vi "Configure Math (Binary Operation).vi"(0 "VISA resource name":refnum<visa-resource-name>, 1 "Enable Math Channel (T:Enable)":bool=TRUE, 2 "Math Operation (12: Add)":i32(ring)=12 items=["Add"=12, "Divide"=13, "Multiply"=14, "Subtract"=15, "Common Mode"=16, "Versus"=17], 5 "Math Channel (0: Function 1)":i32(ring) items=["Function 1", "Function 2", "Function 3", "Function 4", "Function 5", "Function 6", "Function 7", "Function 8", "Function 9", "Function 10", "Function 11", "Function 12", "Function 13", "Function 14", "Function 15", "Function 16"], 7 "Math Operand (1: Channel 1)":i32(ring)=1 items=["Channel 1"=1, "Channel 2"=2, "Channel 3"=3, "Channel 4"=4, "Function 1"=5, "Function 2"=6, "Function 3"=7, "Function 4"=8, "Memory 1"=9, "Memory 2"=10, "Memory 3"=11, "Memory 4"=12, "Differential 1"=61, "Differential 2"=62, "Common 1"=71, "Common 2"=72], 9 "Math Operand 2 (2: Channel 2)":i32(ring)=2 items=["Channel 1"=1, "Channel 2"=2, "Channel 3"=3, "Channel 4"=4, "Function 1"=5, "Function 2"=6, "Function 3"=7, "Function 4"=8, "Memory 1"=9, "Memory 2"=10, "Memory 3"=11, "Memory 4"=12, "Differential 1"=61, "Differential 2"=62, "Common 1"=71, "Common 2"=72], 11 "error in (no error)":errorcluster) -> (4 "VISA resource name out":refnum<visa-resource-name>, 15 "error out":errorcluster)   [LabVIEW 2020, in "Agilent 90000 Series.lvlib"]
doc: "Creates a mathematical expression with two operands."
uses:
  Agilent 90000 Series.lvlib
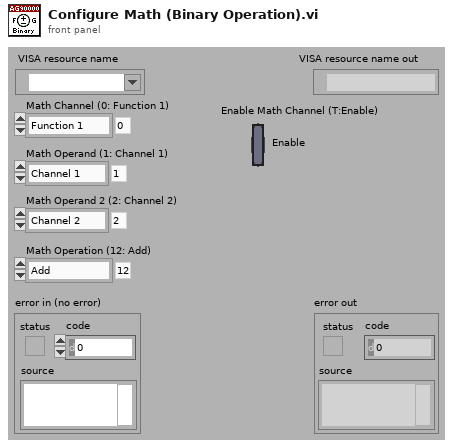
[diagram p1: front panel]
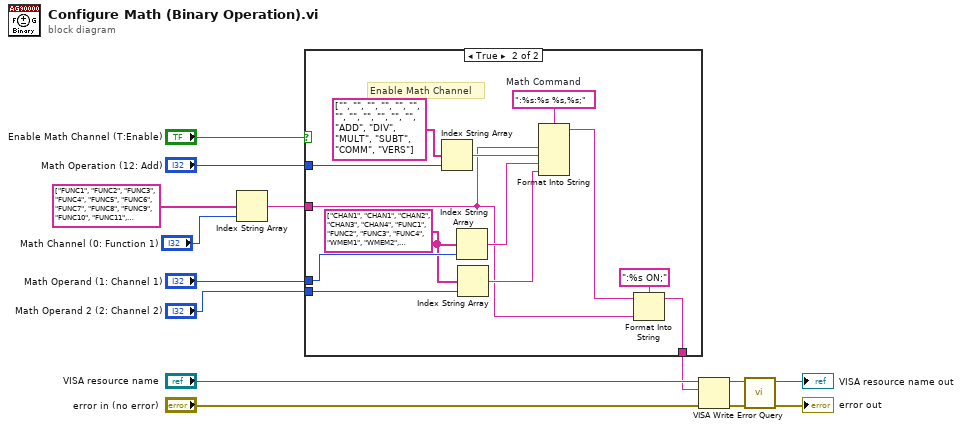
[diagram p0: block diagram]
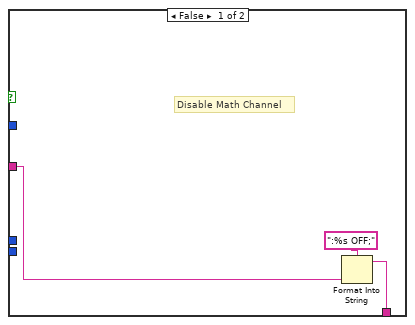
[diagram p2: hidden frame]
diagram:
  n1 = Index String Array(1:"Math Channel (0: Function 1)", 2:string[] ["FUNC1", "FUNC2", "FUNC3", "FUNC4", "FUNC5", "FUNC6", "FUNC7", "FUNC8", "FUNC9", "FUNC10", "FUNC11", "FUNC12", "FUNC13", "FUNC14", "FUNC15", "FUNC16"] ("string array")) -> (0:w7:string)  [unwired: 1 in]
  n2 = case shown="True" "Enable Math Channel (T:Enable)" {
    tunnel: w7 -> [w16 w23]
    tunnel: [w15 w22] -> w6
    tunnel: "Math Operation (12: Add)" -> [_ w21]
    tunnel: "Math Operand (1: Channel 1)" -> [_ w20]
    tunnel: "Math Operand 2 (2: Channel 2)" -> [_ w19]
    frame False {
      # "Disable Math Channel"
      n3 = Format Into String(format string=":%s OFF;", w16) -> (resulting string=w15:string)  [unwired: 2 in, 1 out]
    }
    frame True {
      w18 = string[] ["CHAN1", "CHAN1", "CHAN2", "CHAN3", "CHAN4", "FUNC1", "FUNC2", "FUNC3", "FUNC4", "WMEM1", "WMEM2", "WMEM3", "WMEM4", "AUX", "LINE", "CLOC", "MTR", "MSP", "EQU", "NONE", "DIG0", "DIG1", "DIG2", "DIG3", "DIG4", "DIG5", "DIG6", "DIG7", "DIG8", "DIG9", "DIG10", "DIG11", "DIG12", "DIG13", "DIG14", "DIG15", "", "", "", "", "", "POD1", "POD2", "", "", "", "", "", "", "", "", "BUS1", "BUS2", "BUS3", "BUS4", "", "", "", "", "", "", "DIFF1", "DIFF2", "", "", "", "", "", "", "", "", "COMM3", "COMM4"]
      w29 = ":%s:%s %s,%s;"  # Math Command
      # "Enable Math Channel"
      n4 = Index String Array(1:w21, 2:string[] ["", "", "", "", "", "", "", "", "", "", "", "", "ADD", "DIV", "MULT", "SUBT", "COMM", "VERS"]) -> (0:w28:string)  [unwired: 1 out]
      n5 = Index String Array(1:w20, 2:w18) -> (0:w27:string)  [unwired: 1 in]
      n6 = Index String Array(1:w19, 2:w18) -> (0:w26:string)  [unwired: 1 in]
      n7 = Format Into String(format string=w29, w23, w28, w27, w26) -> (resulting string=w24:string)  [unwired: 2 in, 1 out]
      n8 = Format Into String(format string=":%s ON;", initial string=w24, w23) -> (resulting string=w22:string)  [unwired: 1 in, 1 out]
    }
  }
  n9 = VISA Write(VISA resource name="VISA resource name", write buffer=w6, error in (no error)="error in (no error)") -> (VISA resource name out=w10:refnum<visa-resource-name>, error out=w9:errorcluster)  [unwired: 1 out]
  n10 = call "Error Query.vi"("error in (no error)"=w9, "VISA resource name"=w10) -> ("error out"=→"error out":errorcluster, "VISA resource name out"=→"VISA resource name out":refnum<visa-resource-name>)  [unwired: 8 out]
